vi "AI_test.vi"() -> ()   [LabVIEW 2016]
doc: "이 예제는 DAQmx 디바이스를 사용하여 버퍼있는 전류 측정값을 연속적으로 수집하는 방법을 보여줍니다.\n\n신호를 DAQ 디바이스에 연결하는 방법은 디바이스 문서를 참조하십시오."
uses:
  <vilib>/Utility/error.llb/DialogType.ctl
  <vilib>/DAQmx/read.llb/DAQmx Read (Analog 1D Wfm NChan NSamp).vi
  <vilib>/DAQmx/create/channels.llb/DAQmx Create Channel (AI-Current-Basic).vi
  <vilib>/DAQmx/configure/timing.llb/DAQmx Timing (Sample Clock).vi
  <vilib>/DAQmx/configure/task.llb/DAQmx Configure Logging (TDMS).vi
  <vilib>/DAQmx/configure/trigger.llb/DAQmx Start Trigger (Digital Edge).vi
  <vilib>/DAQmx/configure/trigger.llb/DAQmx Start Trigger (Time).vi
  <vilib>/DAQmx/configure/trigger.llb/DAQmx Start Trigger (Analog Edge).vi
  <vilib>/DAQmx/miscellaneous.llb/DAQmx Fill In Error Info.vi
  <resource>/objmgr/daqmx.rc
panel:
  in  "트리거 타입":T1(tab)
  in  "디지털 시작 트리거 에지":i32(ring)=10280 caption="에지" items=["상승"=10280, "하강"=10171]
  in  "디지털 시작 트리거 소스":tag="/Dev1/PFI0" caption="소스"
  in  "디지털 일시 정지 트리거 일시 정지 시점":i32(ring)=10192 caption="일시 정지 시점" items=["하이"=10192, "로우"=10214]
  in  "디지털 일시 정지 트리거 소스":tag="/Dev1/PFI0" caption="소스"
  in  "아날로그 시작 트리거 레벨":dbl caption="레벨" format="%0.2f"
  in  "아날로그 시작 트리거 히스테리시스":dbl caption="히스테리시스" format="%.2f"
  in  "아날로그 시작 트리거 기울기":i32(ring)=10280 caption="기울기" items=["상승"=10280, "하강"=10171]
  in  "아날로그 시작 트리거 소스":string="APFI0" caption="소스"
  in  "아날로그 일시 정지 트리거 소스":string="APFI0" caption="소스"
  in  "아날로그 일시 정지 트리거 일시 정지 시점":i32(ring)=10093 caption="일시 정지 시점" items=["레벨 이상"=10093, "레벨 이하"=10107]
  in  "아날로그 일시 정지 트리거 레벨":dbl caption="레벨" format="%.2f"
  in  "시점":timestamp
  in  "수동으로\n시간 선택":bool
  in  "분기 값(ohms)":dbl=249.0 format="%0.2f"
  in  "분기 저항":i32(ring)=-1 items=["기본값"=-1, "내부"=10200, "외부"=10167]
  in  "정지":bool
  out "웨이브폼 그래프":waveform(dbl)[](graph)
  in  "TDMS 파일 경로":path
  in  "루프 당 샘플":i32=1000
  in  "샘플 속도":dbl=1000.0
  in  "샘플 클럭 소스":tag="OnboardClock"
  in  "최대 전류 (A)":dbl=0.02
  in  "최소 전류 (A)":dbl
  in  "물리적 채널":tag="Dev1/ai0"
  out "실제 샘플 속도":dbl=1000.0 format="%0.2f"
  in  "로깅 모드":i32(ring)=10231 items=["Off"=10231, "로그 및 읽기"=15842]
  # "채널 셋팅"
  # "수집한 데이터"
  # "타이밍 셋팅"
  # "트리거 셋팅"
  # "로깅 셋팅"
  # "트리거를 활성화하려면, 위의 탭을 선택하고 셋팅을 설정합니다.\n\n일부 하드웨어는 일부 트리거 타입만 지원합니다. 더 자세한 정보는 디바이스 문서를 참조하십시오."
  # "이 트리거 타입은 연속 샘플 타이밍에서 지원되지 않습니다. \n\n지원되는 트리거가 무엇인지에 대한 더 자세한 정보는 디바이스 문서를 참조하십시오."
  # "이 트리거 타입은 연속 샘플 타이밍에서 지원되지 않습니다. \n\n지원되는 트리거가 무엇인지에 대한 더 자세한 정보는 디바이스 문서를 참조하십시오."
  # "시간을 수동으로 설정하지 않으면, 태스크가 10초 후에 시작됩니다."
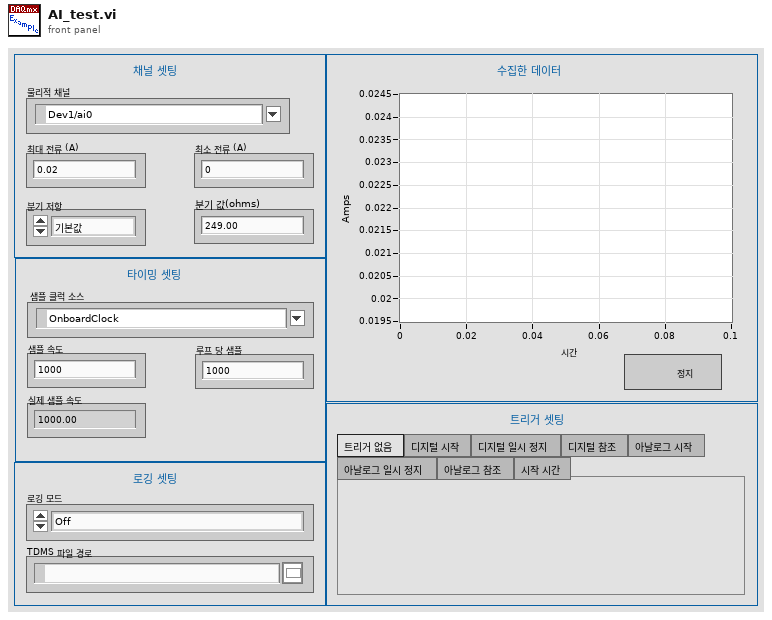
[diagram p1: front panel]
types:
  T1 = enum32{"No Trigger", "Digital Start", "Digital Pause", "Digital Reference", "Analog Start", "Analog Pause", "Analog Reference", "Time Start"}
  T2 = typedef "DialogType.ctl" = u16
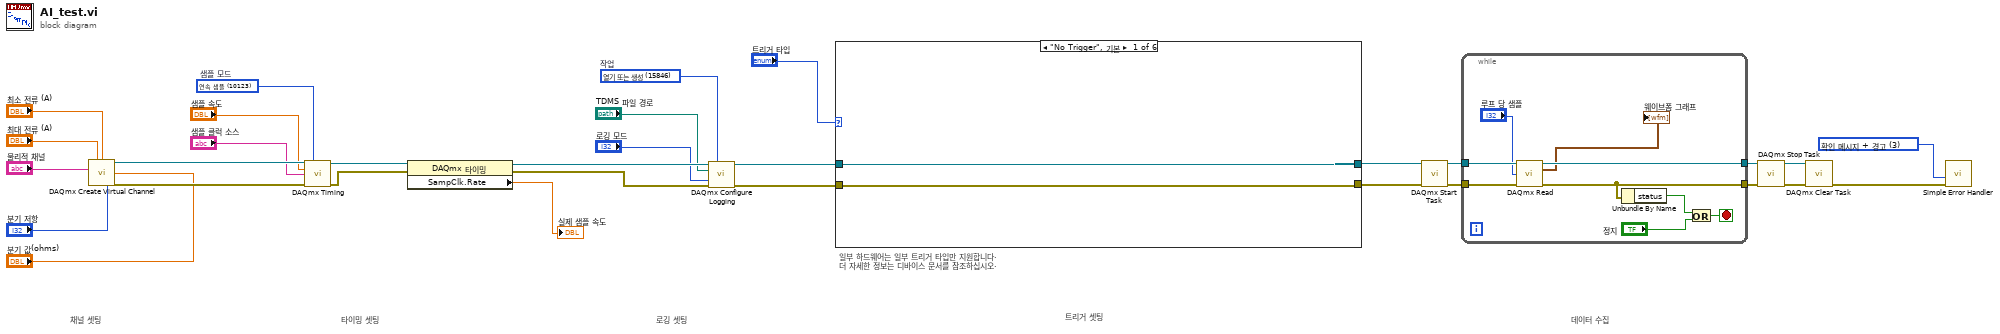
[diagram p0: block diagram]
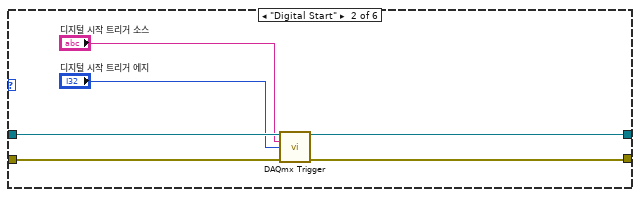
[diagram p2: hidden frame]
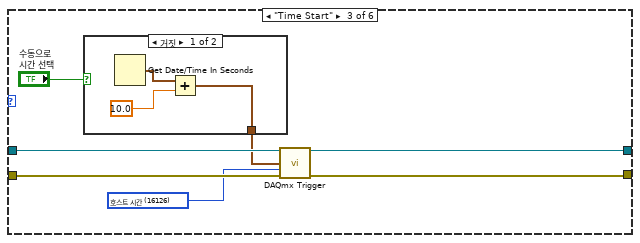
[diagram p3: hidden frame]
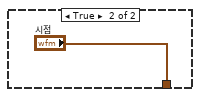
[diagram p4: hidden frame]
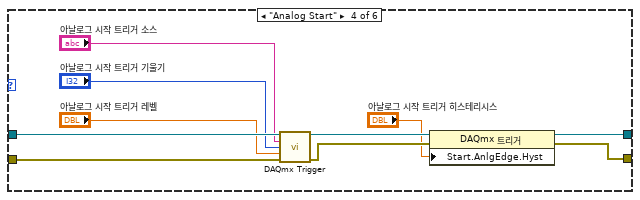
[diagram p5: hidden frame]
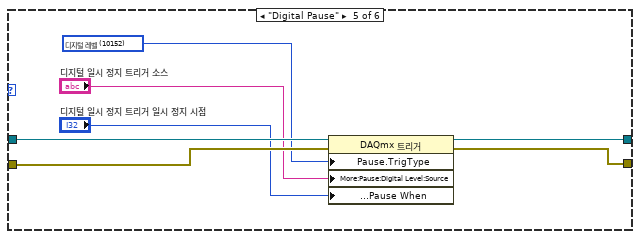
[diagram p6: hidden frame]
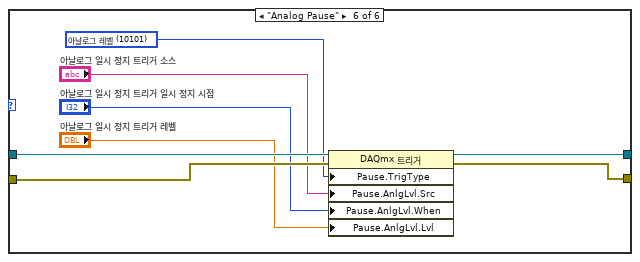
[diagram p7: hidden frame]
diagram:
  w6 = T2 3 items=["대화 상자 없음", "확인 메시지", "메시지 지속 또는 정지", "확인 메시지 + 경고", "지속/정지 + 경고"] ("대화 상자 타입 (확인 메시지:1)")
  w24 = 15846 items=["열기"=10437, "열기 또는 생성"=15846, "생성 또는 대체"=15847, "생성"=15848]  # 작업
  w29 = 10123 items=["유한 샘플"=10178, "연속 샘플"=10123, "하드웨어 타이밍에 의한 단일 포인트"=12522]  # 샘플 모드
  # "트리거 셋팅"
  # "일부 하드웨어는 일부 트리거 타입만 지원합니다.\n더 자세한 정보는 디바이스 문서를 참조하십시오."
  # "데이터 수집"
  # "타이밍 셋팅"
  # "채널 셋팅"
  # "로깅 셋팅"
  n1 = call-poly <vilib>:"DAQmx Create Virtual Channel.vi"("maximum value"="최대 전류 (A)", "minimum value"="최소 전류 (A)", "physical channels"="물리적 채널", "external shunt resistor value"="분기 값(ohms)", "shunt resistor location"="분기 저항") -> ("task out"=w27:refnum<k21>, "error out"=w28:errorcluster)  [unwired: 9 in]
  n2 = call-poly <vilib>:"DAQmx Timing.vi"("task/channels in"=w27, "sample mode"=w29, "rate"="샘플 속도", "source"="샘플 클럭 소스", "error in"=w28) -> ("task out"=w31:refnum<k21>, "error out"=w30:errorcluster)  [unwired: 9 in]
  n3 = property class="DAQmx 타이밍"(reference=w31, error in=w30) -> (reference out=w26:refnum<k21>, error out=w25:errorcluster, "SampClk.Rate"=→"실제 샘플 속도":dbl)
  n4 = call-poly <vilib>:"DAQmx Configure Logging.vi"("task/channels in"=w26, "operation"=w24, "file path"="TDMS 파일 경로", "logging mode"="로깅 모드", "error in"=w25) -> ("task out"=w1:refnum<k21>, "error out"=w4:errorcluster)  [unwired: 9 in]
  n5 = case shown="\"No Trigger\", 기본" "트리거 타입" {
    tunnel: w1 -> [w33 w39 w46 w60 w67 w75]
    tunnel: w4 -> [w32 w38 w45 w59 w64 w72]
    tunnel: [w33 w37 w44 w57 w66 w74] -> w2
    tunnel: [w32 w36 w43 w56 w65 w73] -> w3
    frame "No Trigger", Default {
    }
    frame "Digital Start" {
      n6 = call-poly <vilib>:"DAQmx Trigger.vi"("task/channels in"=w39, "source"="디지털 시작 트리거 소스", "edge"="디지털 시작 트리거 에지", "error in"=w38) -> ("task out"=w37:refnum<k21>, "error out"=w36:errorcluster)  [unwired: 10 in]
    }
    frame "Time Start" {
      w40 = 16126 items=["호스트 시간"=16126, "I/O 디바이스 시간"=16127] ("시간 스케일")
      n7 = case shown="거짓" "수동으로\n시간 선택" {
        tunnel: [w48 "시점"] -> w41
        frame False {
          n8 = Get Date/Time In Seconds() -> (seconds since 1Jan1904=w49:timestamp)
          n9 = Add(x=w49, y=10.0) -> (x+y=w48:timestamp)
        }
        frame True {
        }
      }
      n10 = call-poly <vilib>:"DAQmx Trigger.vi"("task/channels in"=w46, "when"=w41, "timescale"=w40, "error in"=w45) -> ("task out"=w44:refnum<k21>, "error out"=w43:errorcluster)  [unwired: 10 in]
    }
    frame "Analog Start" {
      n11 = call-poly <vilib>:"DAQmx Trigger.vi"("task/channels in"=w60, "source"="아날로그 시작 트리거 소스", "slope"="아날로그 시작 트리거 기울기", "level"="아날로그 시작 트리거 레벨", "error in"=w59) -> ("task out"=w55:refnum<k21>, "error out"=w54:errorcluster)  [unwired: 9 in]
      n12 = property class="DAQmx 트리거"(reference=w55, error in=w54, "Start.AnlgEdge.Hyst"="아날로그 시작 트리거 히스테리시스") -> (reference out=w57:refnum<k21>, error out=w56:errorcluster)
    }
    frame "Digital Pause" {
      w63 = 10152 items=["아날로그 레벨"=10101, "아날로그 윈도우"=10103, "디지털 레벨"=10152, "디지털 패턴"=10398, "없음"=10230] ("일시정지.트리거타입")
      n13 = property class="DAQmx 트리거"(reference=w67, error in=w64, "Pause.TrigType"=w63, "More:Pause:Digital Level:Source"="디지털 일시 정지 트리거 소스", "More:Pause:Digital Level:Pause When"="디지털 일시 정지 트리거 일시 정지 시점") -> (reference out=w66:refnum<k21>, error out=w65:errorcluster)
    }
    frame "Analog Pause" {
      w71 = 10101 items=["아날로그 레벨"=10101, "아날로그 윈도우"=10103, "디지털 레벨"=10152, "디지털 패턴"=10398, "없음"=10230] ("일시정지.트리거타입")
      n14 = property class="DAQmx 트리거"(reference=w75, error in=w72, "Pause.TrigType"=w71, "Pause.AnlgLvl.Src"="아날로그 일시 정지 트리거 소스", "Pause.AnlgLvl.When"="아날로그 일시 정지 트리거 일시 정지 시점", "Pause.AnlgLvl.Lvl"="아날로그 일시 정지 트리거 레벨") -> (reference out=w74:refnum<k21>, error out=w73:errorcluster)
    }
  }
  n15 = call <vilib>:"DAQmx Start Task.vi"("task/channels in"=w2, "error in"=w3) -> ("task out"=w23:refnum<k21>, "error out"=w22:errorcluster)  [unwired: 12 in]
  n16 = while {
    tunnel: w23 -> [w84]
    tunnel: w22 -> [w83]
    tunnel: [w80] -> w9
    tunnel: [w81] -> w10
    stop <- w82 stop-if-true
    n17 = call-poly <vilib>:"DAQmx Read.vi"("task/channels in"=w84, "number of samples per channel"="루프 당 샘플", "error in"=w83) -> ("task out"=w81:refnum<k21>, "data"=→"웨이브폼 그래프":waveform(dbl)[], "error out"=w80:errorcluster)  [unwired: 10 in]
    n18 = Unbundle By Name(w80) -> ("status"=w79:bool)
    n19 = Or(x=w79, y="정지") -> (x .or. y?=w82:bool)
  }
  n20 = call <vilib>:"DAQmx Stop Task.vi"("task/channels in"=w10, "error in"=w9) -> ("task out"=w8:refnum<k21>, "error out"=w7:errorcluster)  [unwired: 12 in]
  n21 = call <vilib>:"DAQmx Clear Task.vi"("task in"=w8, "error in"=w7) -> ("error out"=w21:errorcluster)  [unwired: 13 in]
  n22 = call <vilib>:"Simple Error Handler.vi"("type of dialog (OK msg:1)"=w6, "error in (no error)"=w21) -> ()  [unwired: 3 in, 5 out]
